vi "setTestProcedure.vi"() -> ()   [LabVIEW 2015]
panel:
  in  "stop":bool
  in  "Last inn":bool
  out "Table Control":string[][](table) caption="tabell"
  in  "Time(ms)":dbl=0.9
  in  "Amplitude(kPA)":dbl=20.0
  in  "Frequency(kHz)":dbl=30.0
  in  "Temperature(°C)":dbl=100.0
  in  "Ny Input":bool
  in  "lagre":bool
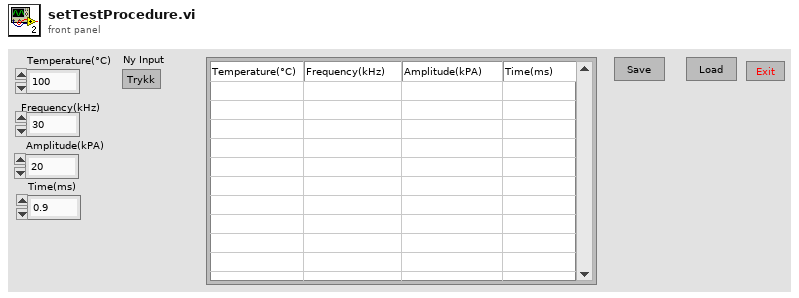
[diagram p1: front panel]
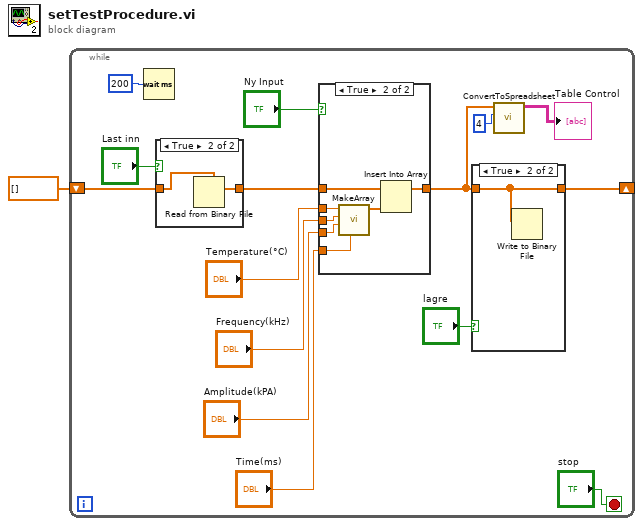
[diagram p0: block diagram]
diagram:
  n1 = while {
    shift-right: [w4] -> _
    shift-left: dbl[] [] ("Array 2") -> [w8]
    stop <- "stop" stop-if-true
    n2 = Wait (ms)(milliseconds to wait=u32 200) -> ()  [unwired: 1 out]
    n3 = case shown="True" "Last inn" {
      tunnel: w8 -> [w19 w21]
      tunnel: [w19 w20] -> w7
      frame False {
      }
      frame True {
        n4 = Read from Binary File(5:w21) -> (2:w20:dbl[])  [unwired: 5 in, 3 out]
      }
    }
    n5 = case shown="True" "Ny Input" {
      tunnel: w7 -> [w22 w23]
      tunnel: "Temperature(°C)" -> [_ w29]
      tunnel: "Frequency(kHz)" -> [_ w28]
      tunnel: "Amplitude(kPA)" -> [_ w27]
      tunnel: "Time(ms)" -> [_ w26]
      tunnel: [w22 w25] -> w3
      frame False {
      }
      frame True {
        n6 = call "MakeArray.vi"("Hviletid(s)"=w26, "Amplitude(kPA)"=w27, "Frekvens(kHz)"=w28, "Temperatur(Celsius)"=w29) -> ("Array"=w24:dbl[])  [unwired: 7 in]
        n7 = Insert Into Array(array=w23, new element=w24) -> (w25:dbl[])  [unwired: 1 in]
      }
    }
    n8 = case shown="True" "lagre" {
      tunnel: w3 -> [w17 w18]
      tunnel: [w17 w18] -> w4
      frame False {
      }
      frame True {
        n9 = Write to Binary File(data=w18) -> ()  [unwired: 5 in, 3 out]
      }
    }
    n10 = call "ConvertToSpreadsheet.vi"("Kolonner"=4, "Array in"=w3) -> ("Array out"=→"Table Control":string[][])  [unwired: 9 in]
  }
